vi "Create 0 Array.vi"(10 "diameter results":dbl[][](array[numeric]), 11 "force results":dbl[][](array[numeric])) -> (3 "Zero array":dbl[][](array[numeric]))   [LabVIEW 2020]
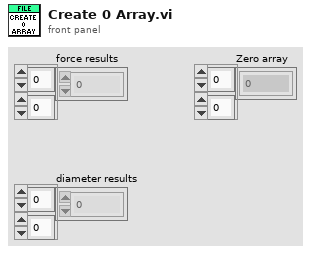
[diagram p1: front panel]
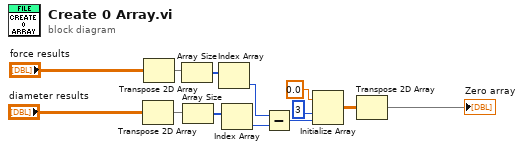
[diagram p0: block diagram]
diagram:
  n1 = Transpose 2D Array(2D array="diameter results") -> (transposed array=w7:dbl[][])
  n2 = Transpose 2D Array(2D array="force results") -> (transposed array=w6:dbl[][])
  n3 = Array Size(array=w6) -> (size(s)=w1:i32[])
  n4 = Array Size(array=w7) -> (size(s)=w2:i32[])
  n5 = Index Array(array=w1) -> (element=w3:i32)  [unwired: 1 in]
  n6 = Index Array(array=w2) -> (element=w4:i32)  [unwired: 1 in]
  n7 = Subtract(x=w3, y=w4) -> (x-y=w10:i32)
  n8 = Initialize Array(0.0 ("element"), 3 ("dimension size"), w10) -> (w11:dbl[][])
  n9 = Transpose 2D Array(2D array=w11) -> (transposed array=→"Zero array":dbl[][])
